vi "Main.vi"() -> ()   [LabVIEW 2020]
doc: "This template is for the Queued Message Handler design pattern.\n\nThe Event Handling Loop generates messages based on user interface actions.\n\nThe Message Handling Loop processes messages generated by the Event Handling Loop, or by other messages. The messages are string values, so new messages can be added easily to the Message Cases case structure in the Message Handling Loop. Each message cluster can also provide an optional value for Message Data, which is a variant that can be converted to whatever message-specific data is required."
uses:
  controls/What animation enum.ctl
  controls/UI Data.ctl
  support/Message Queue/Enqueue Message (Single).vi
  <vilib>/Utility/error.llb/Error Cluster From Error Code.vi
  <vilib>/ErrorRing/Error Ring.xnode
  support/Message Queue/Message Queue.lvlib
  support/User Event - Stop/User Event - Stop.lvlib
panel:
  in  "What animation?":T1
  in  "phase tempo":dbl(knob) scale=-10.0..10.0
  in  "parameter b":i32=1
  out "Display":cluster{"X":dbl[], "Y ":dbl[]}(graph)
  in  "phase":dbl(knob) scale=-180.0..180.0
  in  "parameter a":i32=1
  in  "Exit":bool
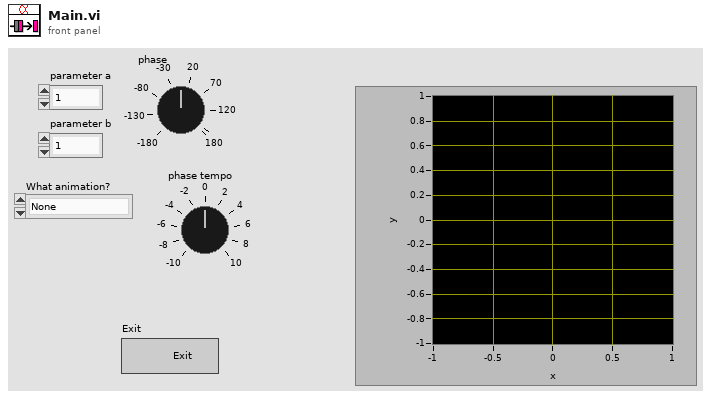
[diagram p1: front panel]
types:
  T1 = typedef "What animation enum.ctl" = enum16{"None", "Phase", "Streak"}
  T2 = typedef "UI Data.ctl" = cluster{"a":i32, "b":i32, "phase(deg)":dbl, "T":i32, "dt":dbl, "T array":dbl[], "curve data":cluster{"X":dbl[], "Y ":dbl[]}, "data for graph":cluster{"X":dbl[], "Y ":dbl[]}, "What animation?":T1, "refresh time (ms)":dbl, "timer (ms)":dbl, "phase change (deg)":dbl}
  T3 = typedef "Message Queue.lvlib/All Message Queues.ctl" = cluster{"UI":refnum<queue>}
  T4 = typedef "animation logic enum 1.ctl" = enum16{"t=0", "t>=max", "0<t<max"}
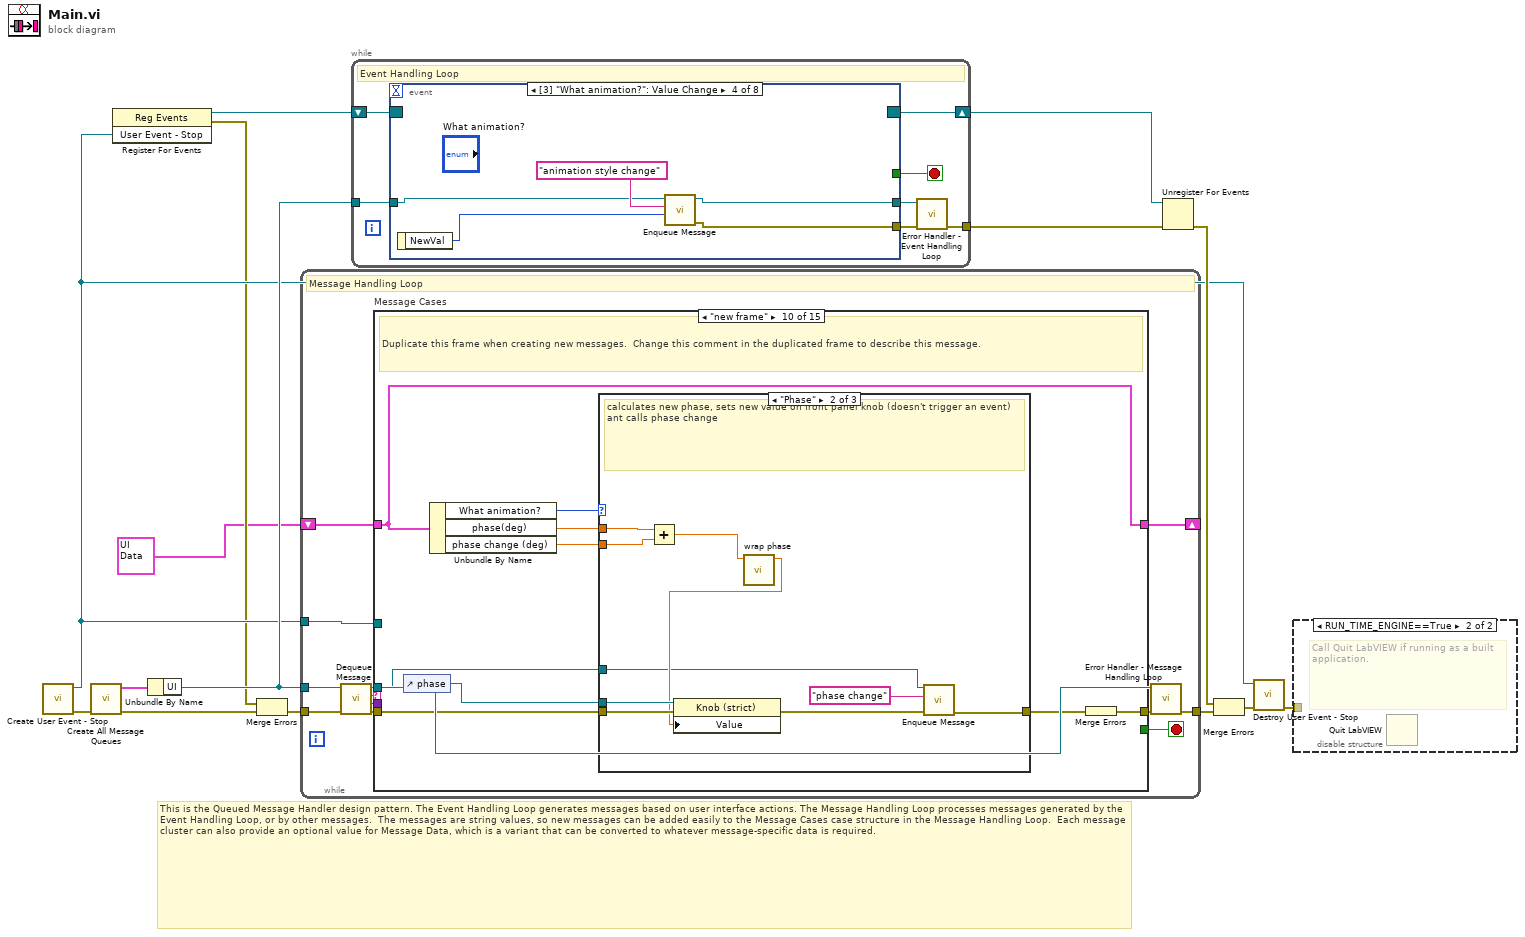
[diagram p0: block diagram]
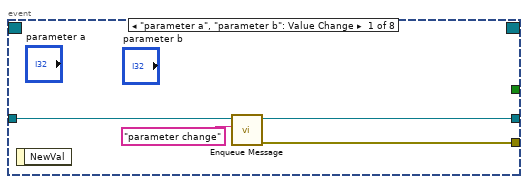
[diagram p3: hidden frame]
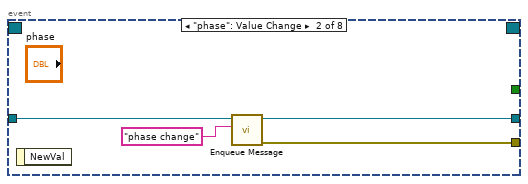
[diagram p4: hidden frame]
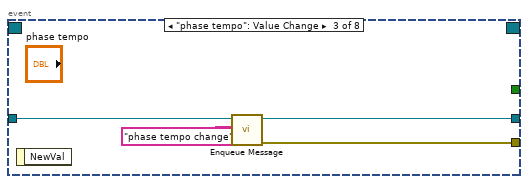
[diagram p5: hidden frame]
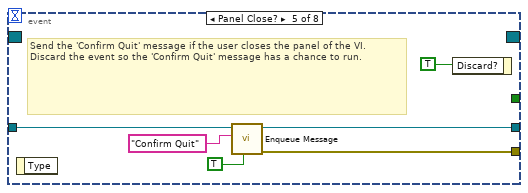
[diagram p6: hidden frame]
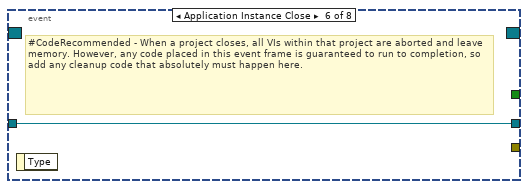
[diagram p7: hidden frame]
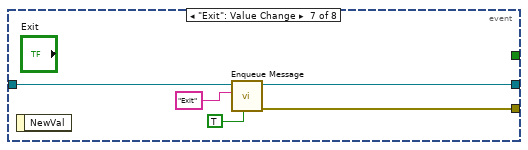
[diagram p8: hidden frame]
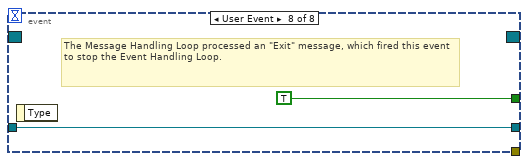
[diagram p9: hidden frame]
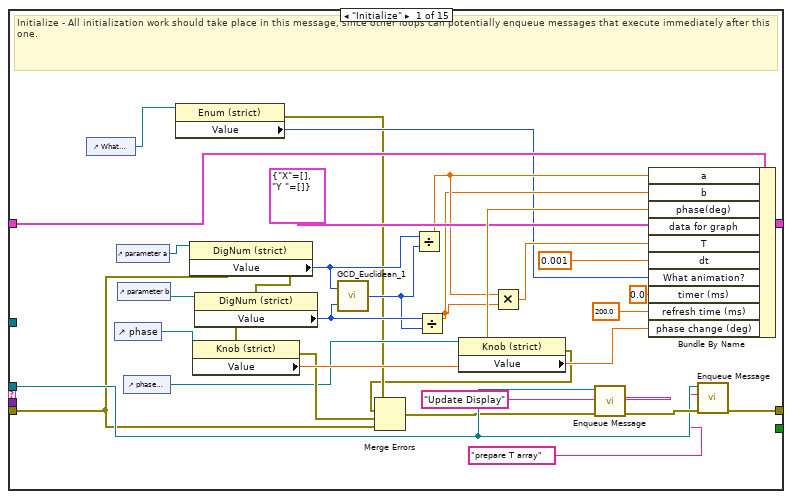
[diagram p10: hidden frame]
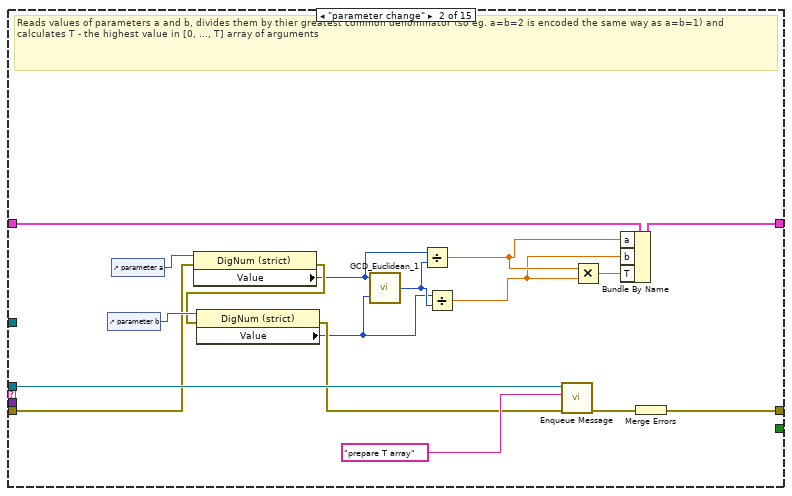
[diagram p11: hidden frame]
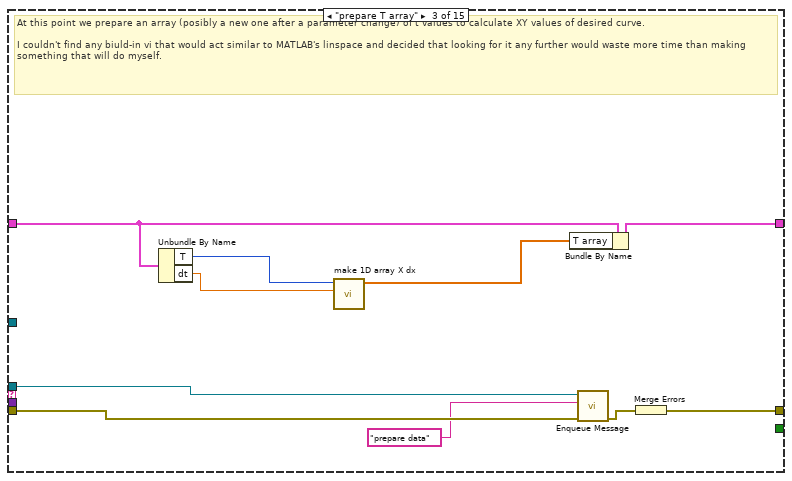
[diagram p12: hidden frame]
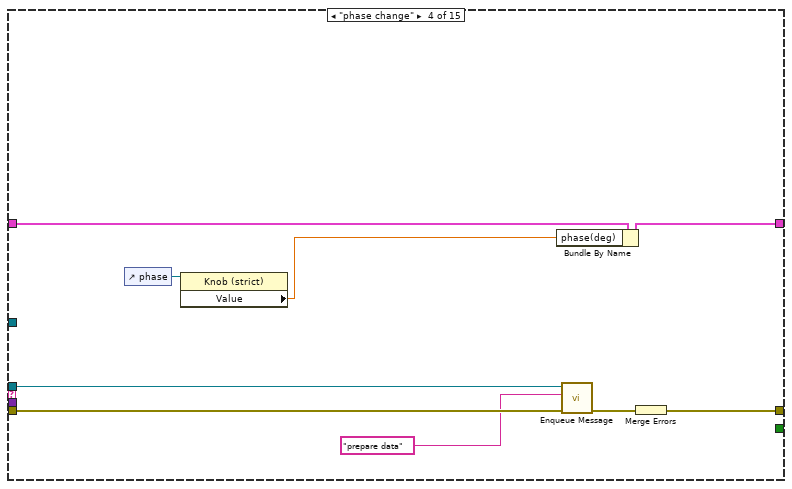
[diagram p13: hidden frame]
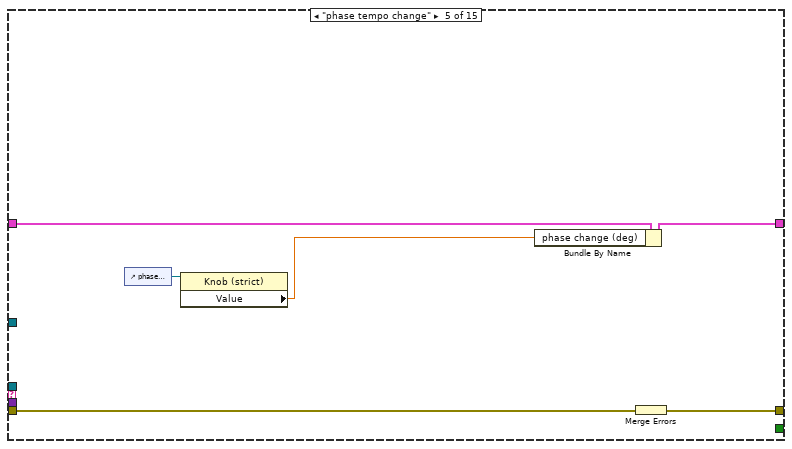
[diagram p14: hidden frame]
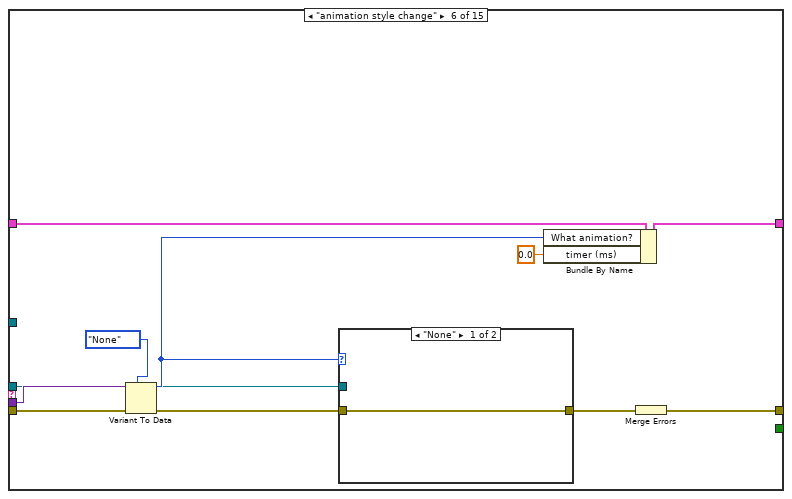
[diagram p15: hidden frame]
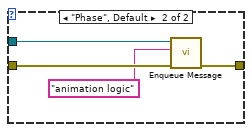
[diagram p16: hidden frame]
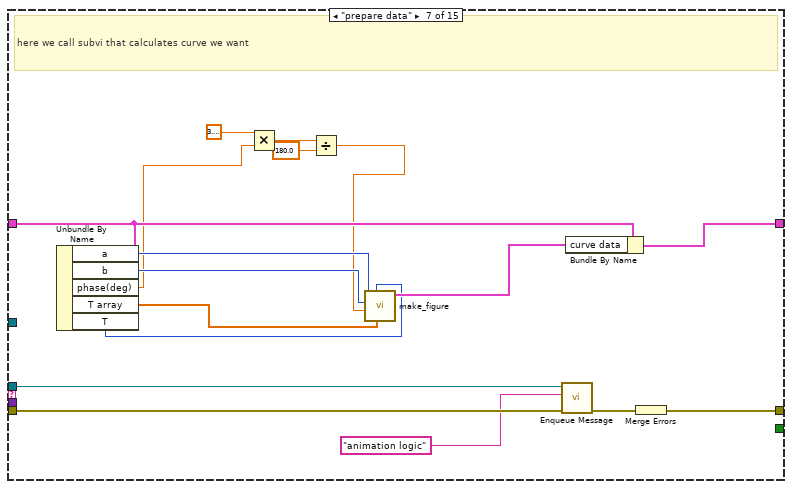
[diagram p17: hidden frame]
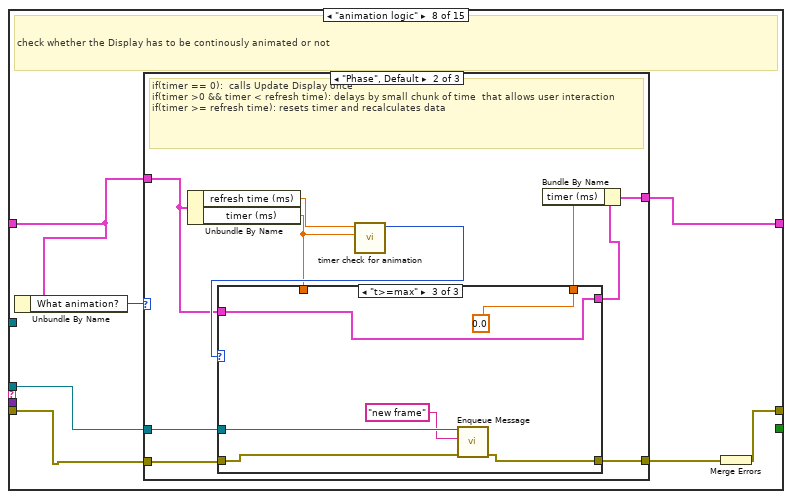
[diagram p18: hidden frame]
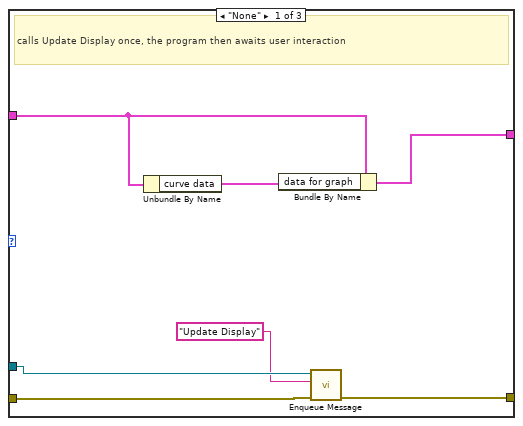
[diagram p19: hidden frame]
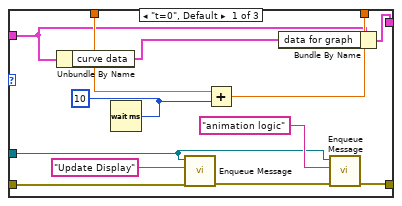
[diagram p20: hidden frame]
diagram:
  # "This is the Queued Message Handler design pattern. The Event Handling Loop generates messages based on user interface actions. The Message Handling Loop processes messages generated by the Event Handling Loop, or by other messages.  The messages are string values, so new messages can be added easily to the Message Cases case structure in the Message Handling Loop.  Each message cluster can also provide an optional value for Message Data, which is a variant that can be converted to whatever message-specific data is required."
  n1 = call "Create User Event - Stop.vi"() -> ("error out"=w11:errorcluster, "User Event - Stop"=w4:refnum<user-event>)  [unwired: 10 in]
  n2 = call "Create All Message Queues.vi"("error in (no error)"=w11) -> ("error out"=w15:errorcluster, "Message Queues out"=w14:T3)  [unwired: 9 in]
  n3 = register-events(w4) -> (reference out=w5:refnum<event-registration>, error out=w2:errorcluster)  [unwired: 2 in]
  n4 = Unbundle By Name(w14) -> ("UI"=w12:refnum<queue>)
  n5 = Merge Errors(w2, w15) -> (w3:errorcluster)
  n6 = while {
    tunnel: w12 -> [w19]
    shift-right: [w26] -> _
    shift-left: T2 {"a"=0, "b"=0, "phase(deg)"=0.0, "T"=0, "dt"=0.0, "T array"=[], "curve data"={"X"=[], "Y "=[]}, "data for graph"={"X"=[], "Y "=[]}, "What animation?"=enum."None", "refresh time (ms)"=0.0, "timer (ms)"=0.0, "phase change (deg)"=0.0} ("UI Data") -> [w27]
    tunnel: w4 -> [w24]
    tunnel: w3 -> [w23]
    tunnel: [w17] -> w13
    stop <- w25 stop-if-true
    # "Message Handling Loop"
    n7 = call "Dequeue Message.vi"("error in (no error)"=w23, "Message Queue"=w19) -> ("error out"=w22:errorcluster, "Message Data"=w20:variant, "Message"=w21:string, "dup Message Queue"=w18:refnum<queue>)  [unwired: 6 in]
    n8 = case "Message Cases" shown="\"new frame\"" w21 {
      selector: w21 -> [_ _ _ _ _ _ _ _ _ _ _ _ _ _ w240]
      tunnel: w18 -> [w44 w73 w78 w92 _ w103 w131 w135 _ w191 _ w221 _ w239 _]
      tunnel: w22 -> [w30 w69 w80 w94 w96 w109 w133 w137 w189 w196 w218 w225 w228 w232 _]
      tunnel: [w45 w75 w86 w95 w101 w112 w134 w141 w190 w199 w212 w223 w226 w235 w241] -> w16
      tunnel: w27 -> [w37 w76 w85 w87 w97 w110 w128 w139 w188 w198 w217 w224 w227 w238 w242]
      tunnel: [w59 w66 w82 w89 w99 w111 w129 w138 w188 w198 w217 w224 w227 w238 w242] -> w26
      tunnel: [_ _ _ _ _ _ _ _ _ _ _ _ _ TRUE _] -> w25
      tunnel: w20 -> [_ _ _ _ _ w108 _ _ _ _ w216 _ _ w229 _]
      tunnel: w24 -> [_ _ _ _ _ _ _ _ _ _ _ _ _ w234 _]
      frame "Initialize" {
        # "Initialize - All initialization work should take place in this message, since other loops can potentially enqueue messages that execute immediately after this one."
        n9 = control-ref of="What animation?"() -> (w33:refnum<vi>)
        n10 = control-ref of="phase"() -> (w55:refnum<vi>)
        n11 = control-ref of="parameter a"() -> (w57:refnum<vi>)
        n12 = control-ref of="parameter b"() -> (w56:refnum<vi>)
        n13 = control-ref of="phase tempo"() -> (w34:refnum<vi>)
        n14 = property class="Enum (strict)"(reference=w33) -> (error out=w29:errorcluster, "Value"=w32:T1)  [unwired: 1 in, 1 out]
        n15 = property class="DigNum (strict)"(reference=w57, error in=w30) -> (error out=w52:errorcluster, "Value"=w49:i32)  [unwired: 1 out]
        n16 = property class="DigNum (strict)"(reference=w56, error in=w52) -> (error out=w51:errorcluster, "Value"=w48:i32)  [unwired: 1 out]
        n17 = property class="Knob (strict)"(reference=w55, error in=w51) -> (error out=w50:errorcluster, "Value"=w54:dbl)  [unwired: 1 out]
        n18 = call "GCD_Euclidean_1.vi"("integer 2"=w48, "integer 1"=w49) -> ("gcd"=w47:i32)
        n19 = Divide(x=w49, y=w47) -> (x/y=w41:dbl)
        n20 = Divide(x=w48, y=w47) -> (x/y=w40:dbl)
        n21 = property class="Knob (strict)"(reference=w34) -> (error out=w28:errorcluster, "Value"=w35:dbl)  [unwired: 1 in, 1 out]
        n22 = Merge Errors(w29, w28, w50, w30) -> (w31:errorcluster)
        n23 = Multiply(x=w41, y=w40) -> (x*y=w42:dbl)
        n24 = call-poly "Enqueue Message.vi"("error in (no error)"=w31, "Message"="Update Display", "Message Queue"=w44) -> ("error out"=w46:errorcluster)  [unwired: 7 in, 1 out]
        n25 = Bundle By Name(cluster=w37, "a"=w41, "b"=w40, "phase(deg)"=w54, "data for graph"=cluster{"X":dbl[], "Y ":dbl[]} {"X"=[], "Y "=[]}, "T"=w42, "dt"=0.001 ("dx"), "What animation?"=w32, "timer (ms)"=0.0, "refresh time (ms)"=200.0, "phase change (deg)"=w35) -> (w59:T2)
        n26 = call-poly "Enqueue Message.vi"("error in (no error)"=w46, "Message"="prepare T array", "Message Queue"=w44) -> ("error out"=w45:errorcluster)  [unwired: 7 in, 1 out]
      }
      frame "parameter change" {
        # "Reads values of parameters a and b, divides them by thier greatest common denominator (so eg. a=b=2 is encoded the same way as a=b=1) and calculates T - the highest value in [0, ..., T] array of arguments"
        n27 = control-ref of="parameter b"() -> (w70:refnum<vi>)
        n28 = control-ref of="parameter a"() -> (w71:refnum<vi>)
        n29 = property class="DigNum (strict)"(reference=w71, error in=w69) -> (error out=w68:errorcluster, "Value"=w63:i32)  [unwired: 1 out]
        n30 = property class="DigNum (strict)"(reference=w70, error in=w68) -> (error out=w67:errorcluster, "Value"=w64:i32)  [unwired: 1 out]
        n31 = call "GCD_Euclidean_1.vi"("integer 2"=w64, "integer 1"=w63) -> ("gcd"=w65:i32)
        n32 = Divide(x=w63, y=w65) -> (x/y=w62:dbl)
        n33 = Divide(x=w64, y=w65) -> (x/y=w61:dbl)
        n34 = call-poly "Enqueue Message.vi"("error in (no error)"=w67, "Message"="prepare T array", "Message Queue"=w73) -> ("error out"=w74:errorcluster)  [unwired: 7 in, 1 out]
        n35 = Multiply(x=w62, y=w61) -> (x*y=w60:dbl)
        n36 = Bundle By Name(cluster=w76, "a"=w62, "b"=w61, "T"=w60) -> (w66:T2)
        n37 = Merge Errors(w74) -> (w75:errorcluster)
      }
      frame "prepare T array" {
        # "At this point we prepare an array (posibly a new one after a parameter change) of t values to calculate XY values of desired curve.\n\nI couldn't find any biuld-in vi that would act similar to MATLAB's linspace and decided that looking for it any further would waste more time than making something that will do myself."
        n38 = Unbundle By Name(w85) -> ("T"=w84:i32, "dt"=w83:dbl)
        n39 = call "make 1D array X dx.vi"("dx"=w83, "X"=w84) -> ("Array"=w81:dbl[])  [unwired: 9 in]
        n40 = Bundle By Name(cluster=w85, "T array"=w81) -> (w82:T2)
        n41 = call-poly "Enqueue Message.vi"("error in (no error)"=w80, "Message"="prepare data", "Message Queue"=w78) -> ("error out"=w79:errorcluster)  [unwired: 7 in, 1 out]
        n42 = Merge Errors(w79) -> (w86:errorcluster)
      }
      frame "phase change" {
        n43 = control-ref of="phase"() -> (w90:refnum<vi>)
        n44 = property class="Knob (strict)"(reference=w90) -> ("Value"=w88:dbl)  [unwired: 1 in, 2 out]
        n45 = Bundle By Name(cluster=w87, "phase(deg)"=w88) -> (w89:T2)
        n46 = call-poly "Enqueue Message.vi"("error in (no error)"=w94, "Message"="prepare data", "Message Queue"=w92) -> ("error out"=w93:errorcluster)  [unwired: 7 in, 1 out]
        n47 = Merge Errors(w93) -> (w95:errorcluster)
      }
      frame "phase tempo change" {
        n48 = control-ref of="phase tempo"() -> (w100:refnum<vi>)
        n49 = property class="Knob (strict)"(reference=w100) -> ("Value"=w98:dbl)  [unwired: 1 in, 2 out]
        n50 = Bundle By Name(cluster=w97, "phase change (deg)"=w98) -> (w99:T2)
        n51 = Merge Errors(w96) -> (w101:errorcluster)
      }
      frame "animation style change" {
        n52 = Variant To Data(error in=w109, type=What_animation_enum."None" ("What animation?"), Variant=w108) -> (data=w106:T1, error out=w105:errorcluster)
        n53 = case shown="\"None\"" w106 {
          tunnel: w105 -> [w113 w117]
          tunnel: [w113 w116] -> w104
          tunnel: w103 -> [_ w115]
          frame "None" {
          }
          frame "Phase", Default {
            n54 = call-poly "Enqueue Message.vi"("error in (no error)"=w117, "Message"="animation logic", "Message Queue"=w115) -> ("error out"=w116:errorcluster)  [unwired: 7 in, 1 out]
          }
        }
        n55 = Bundle By Name(cluster=w110, "What animation?"=w106, "timer (ms)"=0.0) -> (w111:T2)
        n56 = Merge Errors(w104) -> (w112:errorcluster)
      }
      frame "prepare data" {
        # "here we call subvi that calculates curve we want"
        n57 = Unbundle By Name(w128) -> ("a"=w127:i32, "b"=w126:i32, "phase(deg)"=w119:dbl, "T array"=w125:dbl[], "T"=w123:i32)
        n58 = Multiply(x=3.141592653589793, y=w119) -> (x*y=w122:dbl)
        n59 = Divide(x=w122, y=180.0) -> (x/y=w118:dbl)
        n60 = call "make_figure.vi"("T Array"=w125, "T"=w123, "phase (rad)"=w118, "b"=w126, "a"=w127) -> ("data for display"=w124:cluster{dbl[], dbl[]})  [unwired: 6 in]
        n61 = call-poly "Enqueue Message.vi"("error in (no error)"=w133, "Message"="animation logic", "Message Queue"=w131) -> ("error out"=w132:errorcluster)  [unwired: 7 in, 1 out]
        n62 = Bundle By Name(cluster=w128, "curve data"=w124) -> (w129:T2)
        n63 = Merge Errors(w132) -> (w134:errorcluster)
      }
      frame "animation logic" {
        # "check whether the Display has to be continously animated or not"
        n64 = Unbundle By Name(w139) -> ("What animation?"=w140:T1)
        n65 = case shown="\"Phase\", Default" w140 {
          tunnel: w139 -> [w148 w150 w185]
          tunnel: [w147 w157 w185] -> w138
          tunnel: w137 -> [w145 w154 w186]
          tunnel: [w144 w153 w186] -> w136
          tunnel: w135 -> [w143 w152 _]
          frame "None" {
            # "calls Update Display once, the program then awaits user interaction"
            n66 = Unbundle By Name(w148) -> ("curve data"=w146:cluster{"X":dbl[], "Y ":dbl[]})
            n67 = Bundle By Name(cluster=w148, "data for graph"=w146) -> (w147:T2)
            n68 = call-poly "Enqueue Message.vi"("error in (no error)"=w145, "Message"="Update Display", "Message Queue"=w143) -> ("error out"=w144:errorcluster)  [unwired: 7 in, 1 out]
          }
          frame "Phase", Default {
            # "if(timer == 0):  calls Update Display once \nif(timer >0 && timer < refresh time): delays by small chunk of time  that allows user interaction \nif(timer >= refresh time): resets timer and recalculates data"
            n69 = Unbundle By Name(w150) -> ("refresh time (ms)"=w158:dbl, "timer (ms)"=w151:dbl)
            n70 = call "timer check for animation.vi"("timer (ms)"=w151, "refresh time (ms)"=w158) -> ("Enum"=w155:T4)  [unwired: 9 in]
            n71 = case shown="\"t>=max\"" w155 {
              tunnel: w151 -> [w169 w178 _]
              tunnel: [w168 w177 0.0] -> w156
              tunnel: [w165 w174 w182] -> w153
              tunnel: w154 -> [w167 w175 w183]
              tunnel: w152 -> [w162 w172 w181]
              tunnel: w150 -> [w161 w171 w179]
              tunnel: [w159 w171 w179] -> w149
              frame "t=0", Default {
                w170 = u32 10 ("milliseconds to wait")
                n72 = Unbundle By Name(w161) -> ("curve data"=w160:cluster{"X":dbl[], "Y ":dbl[]})
                n73 = Wait (ms)(milliseconds to wait=w170) -> ()  [unwired: 1 out]
                n74 = call-poly "Enqueue Message.vi"("error in (no error)"=w167, "Message"="Update Display", "Message Queue"=w162) -> ("error out"=w166:errorcluster)  [unwired: 7 in, 1 out]
                n75 = Add(x=w169, y=w170) -> (x+y=w168:dbl)
                n76 = Bundle By Name(cluster=w161, "data for graph"=w160) -> (w159:T2)
                n77 = call-poly "Enqueue Message.vi"("error in (no error)"=w166, "Message"="animation logic", "Message Queue"=w162) -> ("error out"=w165:errorcluster)  [unwired: 7 in, 1 out]
              }
              frame "0<t<max" {
                w176 = u32 10 ("milliseconds to wait")
                n78 = Wait (ms)(milliseconds to wait=w176) -> ()  [unwired: 1 out]
                n79 = Add(x=w178, y=w176) -> (x+y=w177:dbl)
                n80 = call-poly "Enqueue Message.vi"("error in (no error)"=w175, "Message"="animation logic", "Message Queue"=w172) -> ("error out"=w174:errorcluster)  [unwired: 7 in, 1 out]
              }
              frame "t>=max" {
                n81 = call-poly "Enqueue Message.vi"("error in (no error)"=w183, "Message"="new frame", "Message Queue"=w181) -> ("error out"=w182:errorcluster)  [unwired: 7 in, 1 out]
              }
            }
            n82 = Bundle By Name(cluster=w149, "timer (ms)"=w156) -> (w157:T2)
          }
          frame "Streak" {
            # "#todo"
          }
        }
        n83 = Merge Errors(w136) -> (w141:errorcluster)
      }
      frame "Update Display" {
        # "Update Display - reads 2D array that holds points of the calculated curve and sends it to the Display"
        n84 = Unbundle By Name(w188) -> ("data for graph"=→"Display":cluster{"X":dbl[], "Y ":dbl[]})
        n85 = Merge Errors(w189) -> (w190:errorcluster)
      }
      frame "new frame" {
        # "Duplicate this frame when creating new messages.  Change this comment in the duplicated frame to describe this message."
        n86 = control-ref of="phase"() -> (w194:refnum<vi>)
        n87 = Unbundle By Name(w198) -> ("What animation?"=w195:T1, "phase(deg)"=w193:dbl, "phase change (deg)"=w192:dbl)
        n88 = case shown="\"Phase\"" w195 {
          tunnel: [w200 w203 w211] -> w197
          tunnel: w196 -> [w200 w209 w211]
          tunnel: w194 -> [_ w210 _]
          tunnel: w193 -> [_ w208 _]
          tunnel: w192 -> [_ w207 _]
          tunnel: w191 -> [_ w202 _]
          frame "None", Default {
          }
          frame "Phase" {
            # "calculates new phase, sets new value on front panel knob (doesn't trigger an event) ant calls phase change"
            n89 = Add(x=w208, y=w207) -> (x+y=w206:dbl)
            n90 = call "wrap phase.vi"("phase in (deg)"=w206) -> ("phase out (deg)"=w205:dbl)  [unwired: 10 in]
            n91 = property class="Knob (strict)"(reference=w210, error in=w209, "Value"=w205) -> (error out=w204:errorcluster)  [unwired: 1 out]
            n92 = call-poly "Enqueue Message.vi"("error in (no error)"=w204, "Message"="phase change", "Message Queue"=w202) -> ("error out"=w203:errorcluster)  [unwired: 7 in, 1 out]
          }
          frame "Streak" {
          }
        }
        n93 = Merge Errors(w197) -> (w199:errorcluster)
      }
      frame "Error" {
        # "#CodeRecommended - If you ever change the name of this \"Error\" message, you'll need to update the name in the Check Loop Error.vi as well."
        # "#CodeRecommended - Consider creating a system for logging errors in some way. These errors are for notification purposes only. Handling of specific errors should be performed in the message frames that generated the error."
        # "Error - Display an error dialog. This message is sent by the \"Error Handler\" VIs at the end of other loops in this application."
        n94 = Variant To Data(error in=w218, type=errorcluster {"status"=FALSE, "code"=0, "source"=""} ("error constant"), Variant=w216) -> (data=w214:errorcluster, error out=w213:errorcluster)
        n95 = call <vilib>:"Simple Error Handler.vi"("error in (no error)"=w214) -> ()  [unwired: 4 in, 5 out]
        n96 = Merge Errors(w213) -> (w212:errorcluster)
      }
      frame "Confirm Quit" {
        # "#CodeNeeded - If you want to provide an \"Are you sure\" dialog (or some other notification) before the application exits, place that code here. This message is typically sent from a Panel Close? event."
        # "Confirm Quit - Message that can confirm whether or not the user wants to exit the application."
        n97 = call-poly "Enqueue Message.vi"("Priority Message? (F)"=TRUE, "error in (no error)"=w225, "Message"="Exit", "Message Queue"=w221) -> ("error out"=w222:errorcluster)  [unwired: 6 in, 1 out]
        n98 = Merge Errors(w222) -> (w223:errorcluster)
      }
      frame "---Copy This Frame---" {
        # "Duplicate this frame when creating new messages.  Change this comment in the duplicated frame to describe this message."
        n99 = Merge Errors(w228) -> (w226:errorcluster)
      }
      frame "Exit" {
        # "Stop the VI"
        # "Release the message queue reference"
        # "#CodeNeeded - Add any required cleanup code here. Note that if 'Exit' was called as a result of an error, an error dialog will be displayed. Add any custom error handling for an 'Exit' condition here as well."
        # "Exit - Exit the application."
        n100 = Variant To Data(type=errorcluster {"status"=FALSE, "code"=0, "source"=""} ("error constant"), Variant=w229) -> (data=w230:errorcluster)  [unwired: 1 in, 1 out]
        n101 = call <vilib>:"Simple Error Handler.vi"("error in (no error)"=w230) -> ()  [unwired: 4 in, 5 out]
        n102 = call "Fire User Event - Stop.vi"("User Event - Stop"=w234) -> ("error out"=w233:errorcluster)  [unwired: 10 in]
        n103 = Release Queue(queue=w239, error in (no error)=w232) -> (error out=w236:errorcluster)  [unwired: 1 in, 2 out]
        n104 = Merge Errors(w233, w236) -> (w235:errorcluster)
      }
      frame Default {
        # "'Default' case only runs if there is a message that isn't defined in any of the other cases.  Output a programming error."
        n105 = xnode "Error Ring"("parameter 0"=w240) -> ("error out"=w241:errorcluster)
      }
    }
    n106 = call "Error Handler - Message Handling Loop.vi"("error in (no error)"=w16, "Message Queue"=w18) -> ("dup error in"=w17:errorcluster)  [unwired: 8 in, 1 out]
  }
  n107 = while {
    tunnel: w12 -> [w256]
    shift-right: [w254] -> w8
    shift-left: w5 -> [w255]
    tunnel: [w250] -> w6
    stop <- w252 stop-if-true
    # "Event Handling Loop"
    n108 = event shown="[3] \"What animation?\": Value Change" {
      selector: w255 -> [_ _ _ _ _ _ _ _]
      dyn-events: [_ _ _ _ _ _ _ _] -> w254
      timeout: _ -> [_ _ _ _ _ _ _ _]
      tunnel: [_ _ _ _ _ _ _ TRUE ("Discard?")] -> w252
      tunnel: w256 -> [w260 w264 w268 w272 w278 w280 w285 w287]
      tunnel: [w257 w261 w265 w270 w277 _ w284 _] -> w253
      tunnel: [w259 w263 w267 w271 w276 w280 w283 w287] -> w251
      event "parameter a", "parameter b": Value Change {
        n109 = event-data() -> ()  [unwired: 1 in, 1 out]
        n110 = call-poly "Enqueue Message.vi"("Message"="parameter change", "Message Queue"=w260) -> ("error out"=w257:errorcluster, "dup Message Queue"=w259:refnum<queue>)  [unwired: 8 in]
      }
      event "phase": Value Change {
        n111 = event-data() -> ()  [unwired: 1 in, 1 out]
        n112 = call-poly "Enqueue Message.vi"("Message"="phase change", "Message Queue"=w264) -> ("error out"=w261:errorcluster, "dup Message Queue"=w263:refnum<queue>)  [unwired: 8 in]
      }
      event "phase tempo": Value Change {
        n113 = event-data() -> ()  [unwired: 1 in, 1 out]
        n114 = call-poly "Enqueue Message.vi"("Message"="phase tempo change", "Message Queue"=w268) -> ("error out"=w265:errorcluster, "dup Message Queue"=w267:refnum<queue>)  [unwired: 8 in]
      }
      event Value Change {
        n115 = event-data() -> ("NewVal"=w269:T1)  [unwired: 1 in]
        n116 = call-poly "Enqueue Message.vi"("Message Data"=w269, "Message"="animation style change", "Message Queue"=w272) -> ("error out"=w270:errorcluster, "dup Message Queue"=w271:refnum<queue>)  [unwired: 7 in]
      }
      event Panel Close? {
        # "Send the 'Confirm Quit' message if the user closes the panel of the VI. Discard the event so the 'Confirm Quit' message has a chance to run."
        n117 = event-data() -> ()  [unwired: 1 in, 1 out]
        n118 = call-poly "Enqueue Message.vi"("Priority Message? (F)"=TRUE, "Message"="Confirm Quit", "Message Queue"=w278) -> ("error out"=w277:errorcluster, "dup Message Queue"=w276:refnum<queue>)  [unwired: 7 in]
        n119 = event-data("Discard?"=TRUE) -> ()  [unwired: 1 in, 1 out]
      }
      event Application Instance Close {
        # "#CodeRecommended - When a project closes, all VIs within that project are aborted and leave memory. However, any code placed in this event frame is guaranteed to run to completion, so add any cleanup code that absolutely must happen here."
        n120 = event-data() -> ()  [unwired: 1 in, 1 out]
      }
      event "Exit": Value Change {
        n121 = event-data() -> ()  [unwired: 1 in, 1 out]
        n122 = call-poly "Enqueue Message.vi"("Priority Message? (F)"=TRUE, "Message"="Exit", "Message Queue"=w285) -> ("error out"=w284:errorcluster, "dup Message Queue"=w283:refnum<queue>)  [unwired: 7 in]
      }
      event User Event {
        # "The Message Handling Loop processed an \"Exit\" message, which fired this event to stop the Event Handling Loop."
        n123 = event-data() -> ()  [unwired: 1 in, 1 out]
      }
    }
    n124 = call "Error Handler - Event Handling Loop.vi"("error in (no error)"=w253, "Message Queue"=w251) -> ("dup error in"=w250:errorcluster)  [unwired: 8 in, 1 out]
  }
  n125 = Unregister For Events(event registration refnum=w8, error in=w6) -> (error out=w9:errorcluster)
  n126 = Merge Errors(w9, w13) -> (w10:errorcluster)
  n127 = call "Destroy User Event - Stop.vi"("error in (no error)"=w10, "User Event - Stop"=w4) -> ("error out"=w7:errorcluster)  [unwired: 9 in]
  n128 = disable-structure shown="RUN_TIME_ENGINE==True" {
    disable-tunnel: w7 -> [_ _]
    frame condition #0 (active) {
    }
    frame condition #1 {
      # "Call Quit LabVIEW if running as a built application."
      n129 = Quit LabVIEW() -> ()  [unwired: 1 in]
    }
  }
